vi "GetExternalInterfaces.vi"(8 "ErrorIn":errorcluster, 11 "ObjectIn":refnum<class "BusAuthorizationUpdated.lvclass">) -> (0 "ErrorOut":errorcluster, 2 "ExternalInterfaces":T1[](array[typedef]), 3 "ObjectOut":refnum<class "BusAuthorizationUpdated.lvclass">)   [LabVIEW 2021, in "BusAuthorizationUpdated.lvclass"]
uses:
  BusAuthorizationUpdated.lvclass
  .Externals/Library_TAF_Support/ClusterArrayConversion/BundledArray.ctl
  BusAuthorizationUpdated.lvclass/BusAuthorizationUpdated.ctl
  .Externals/Library_TAF_BusBase/BusBase/BusBase/BusBase.lvclass
  .Externals/Interface_TAF_AutorizationUpdated/IAuthorizationUpdated/IAuthorizationUpdated.lvclass
  .Externals/Library_TAF_Support/ClusterArrayConversion/ClusterArrayConversion.lvlib
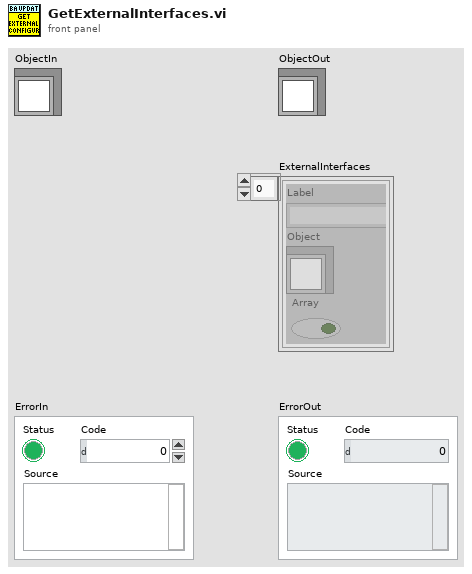
[diagram p1: front panel]
types:
  T1 = typedef "ClusterArrayConversion.lvlib/BundledArray.ctl" = cluster{"Label":string, "Object":refnum<class>, "Array":bool}
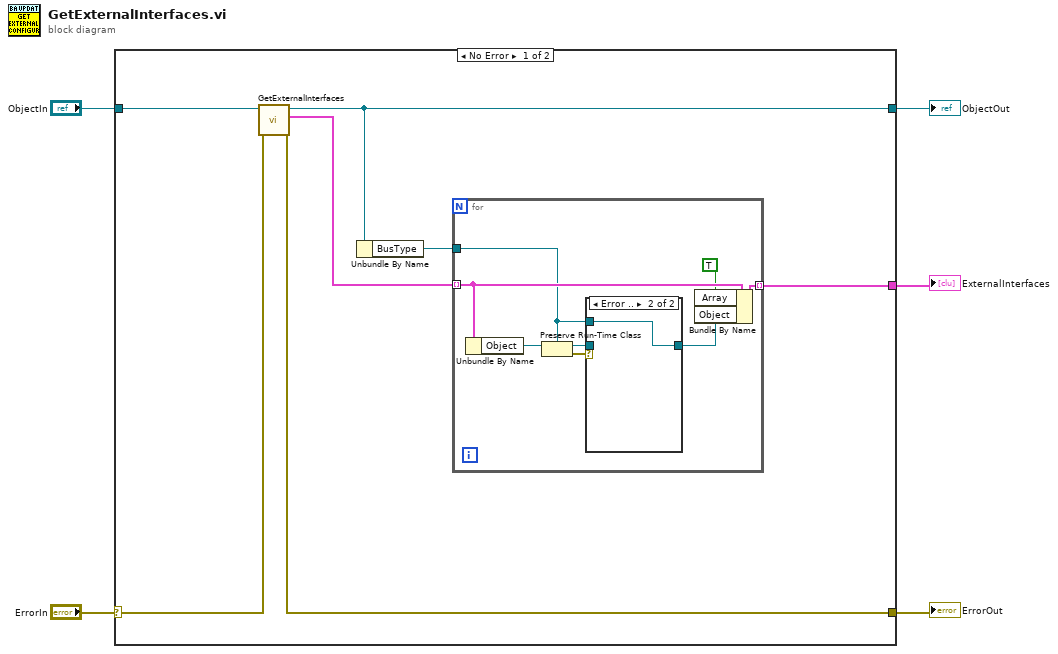
[diagram p0: block diagram]
diagram:
  n1 = case shown="No Error" "ErrorIn" {
    selector: "ErrorIn" -> [w12 w24]
    tunnel: [w11 w24] -> w4
    tunnel: [w9 w23] -> w2
    tunnel: "ObjectIn" -> [w10 w23]
    tunnel: [w6 _] -> w1
    frame No Error {
      n2 = call-parent "GetExternalInterfaces.vi"("ErrorIn"=w12, "ReferenceIn"=w10) -> ("ErrorOut"=w11:errorcluster, "ExternalInterfaces"=w8:T1[], "ReferenceOut"=w9:refnum<class "BusAuthorizationUpdated.lvclass">)  [unwired: 7 in]
      n3 = Unbundle By Name(w9) -> ("BusType"=w7:refnum<class "IAuthorizationUpdated.lvclass">)
      n4 = for {
        tunnel: w8 -> [w17] mode=indexing
        tunnel: w7 -> [w14]
        tunnel: [w15] -> w6 mode=indexing
        n5 = Unbundle By Name(w17) -> ("Object"=w19:refnum<class>)
        n6 = Preserve Run-Time Class(object in=w19, 2:w14) -> (object out=w18:refnum<class "IAuthorizationUpdated.lvclass">, error out=w20:errorcluster)  [unwired: 1 in]
        n7 = case shown="Error .." w20 {
          tunnel: [w21 w22] -> w16
          tunnel: w18 -> [w21 _]
          tunnel: w14 -> [_ w22]
          frame No Error {
          }
          frame Error {
          }
        }
        n8 = Bundle By Name(cluster=w17, "Array"=TRUE, "Object"=w16) -> (w15:T1)
      }
    }
    frame Error {
    }
  }
  "ErrorOut" <- w4
  "ObjectOut" <- w2
  "ExternalInterfaces" <- w1
